vi "Get Item IO.vi"(8 "error in (no error)":errorcluster, 10 "Item Type":enum16{"RSI Module", "User Variables"}(ring), 11 "Item Ref in":T3 format="%.0x") -> (0 "error out":errorcluster, 1 "Output Data":T9 {"BD Refs"."Data Reference" format="%.0x"}, 2 "Input Data":T6 {"BD Refs"."Data Reference" format="%.0x"}, 3 "Item Ref out":T3 format="%.0x", 4 "Mixed IO":T1, 5 "To FPGA":T2[](array[typedef]) {"VS ref" format="%.0x"}, 7 "From FPGA":T2[](array[typedef]) {"VS ref" format="%.0x"})   [LabVIEW 2016, in "Scan Engine Custom Device.lvlib"]
uses:
  Scan Engine Custom Device.lvlib
  Type Defs/Output Data.ctl
  <vilib>/NI Veristand/Custom Device API/Block Data Reference.ctl
  <vilib>/NI Veristand/Custom Device API/Data Reference.ctl
  Type Defs/Input Data.ctl
  <vilib>/NI Veristand/Custom Device API/Custom Device Item Ref.ctl
  Type Defs/UDV Data.ctl
  Type Defs/UDV Data Type.ctl
  Type Defs/FXP Config.ctl
  Type Defs/Mixed IO.ctl
  Type Defs/Data Ref FGV Command.ctl
  <vilib>/NI Veristand/Custom Device API/Custom Device API.lvlib
  <vilib>/NI_Real-Time Target Support.lvlib
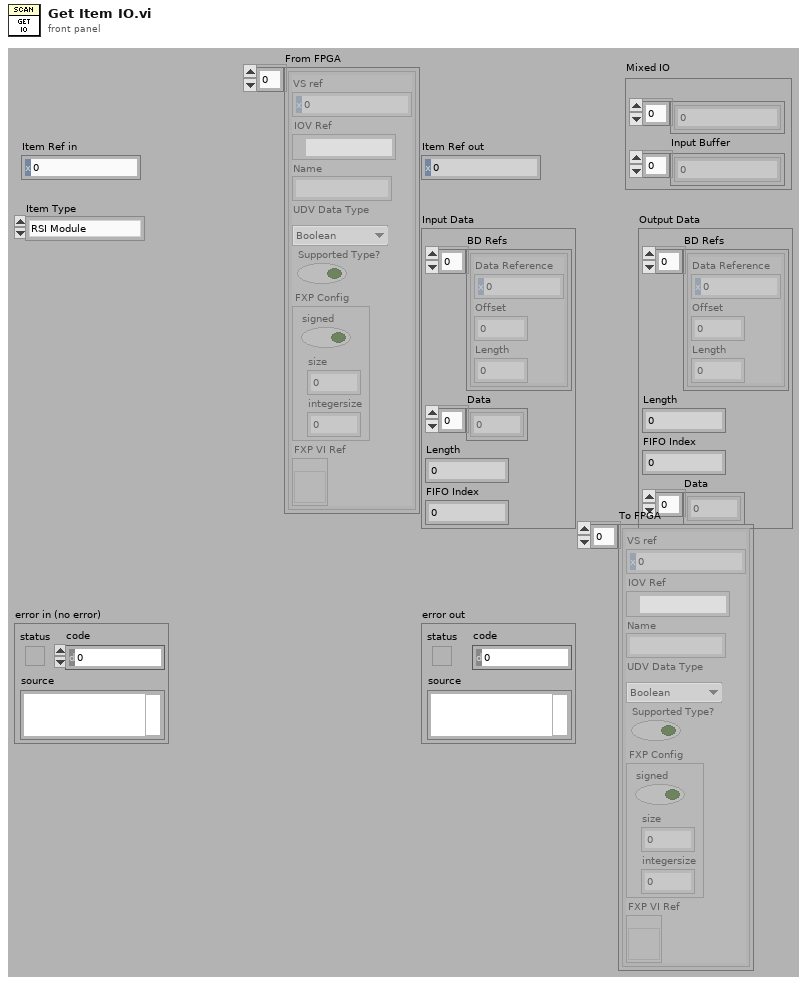
[diagram p1: front panel]
types:
  T1 = typedef "Scan Engine Custom Device.lvlib/Mixed IO.ctl" = cluster{"Input Channel Indices":i32[], "Input Buffer":dbl[]}
  T2 = typedef "Scan Engine Custom Device.lvlib/UDV Data.ctl" = cluster{"VS ref":T3, "IOV Ref":refnum<k21>, "Name":string, "UDV Data Type":T4, "Supported Type?":bool, "FXP Config":T5, "FXP VI Ref":refnum<vi>}
  T3 = typedef "Custom Device API.lvlib/Custom Device Item Ref.ctl" = u64
  T4 = typedef "Scan Engine Custom Device.lvlib/UDV Data Type.ctl" = enum16{"Boolean", "Fixed Point", "Int8", "Int16", "Int32", "Int64", "U32 Bit Field", "UInt8", "UInt16", "UInt32", "UInt64", "Other"}
  T5 = typedef "Scan Engine Custom Device.lvlib/FXP Config.ctl" = cluster{"signed":bool, "size":u32, "integersize":i32}
  T6 = typedef "Scan Engine Custom Device.lvlib/Input Data.ctl" = cluster{"BD Refs":T7[], "Data":dbl[], "Length":i32, "FIFO Index":i32}
  T7 = typedef "Custom Device API.lvlib/Block Data Reference.ctl" = cluster{"Data Reference":T8, "Offset":u64, "Length":u64}
  T8 = typedef "Custom Device API.lvlib/Data Reference.ctl" = i32
  T9 = typedef "Scan Engine Custom Device.lvlib/Output Data.ctl" = cluster{"BD Refs":T7[], "Length":i32, "FIFO Index":i32, "Data":dbl[]}
  T10 = typedef "Scan Engine Custom Device.lvlib/Data Ref FGV Command.ctl" = enum16{"Intialize", "Get", "Update"}
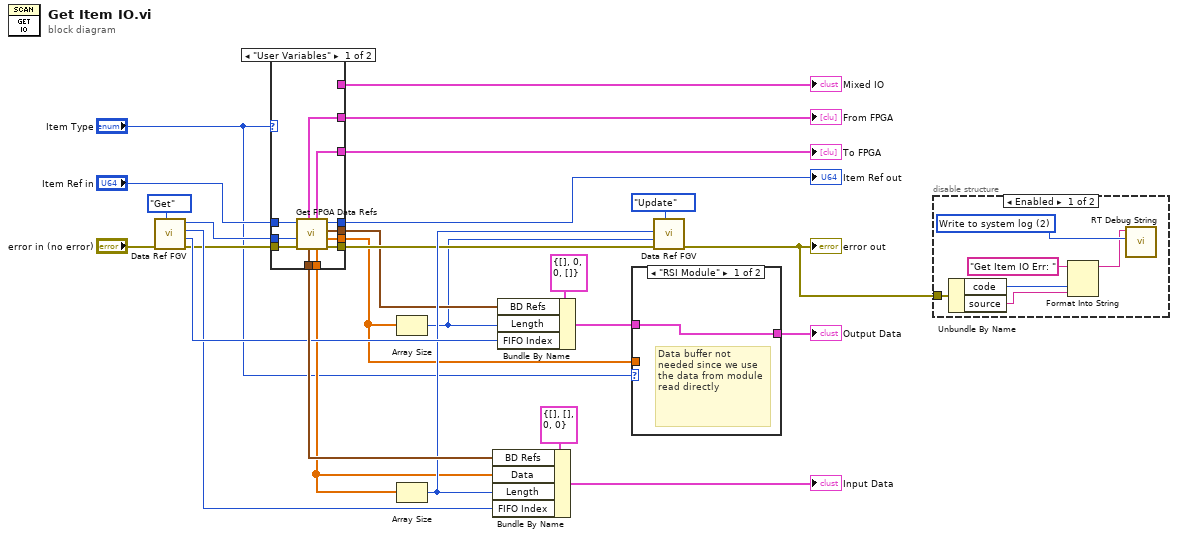
[diagram p0: block diagram]
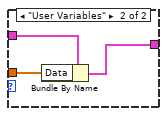
[diagram p3: hidden frame]
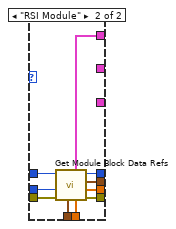
[diagram p4: hidden frame]
diagram:
  n1 = call "Data Ref FGV.vi"("Command"=Data_Ref_FGV_Command."Get", "error in (no error)"="error in (no error)") -> ("error out"=w17:errorcluster, "Output FIFO Index / Length"=w22:i32, "Input FIFO Index / Length"=w21:i32, "Device Ref out"=w12:T3)  [unwired: 6 in]
  n2 = case shown="\"User Variables\"" "Item Type" {
    tunnel: [w33 w47] -> w9
    tunnel: [w34 w46] -> w23
    tunnel: [w32 w45] -> w18
    tunnel: w17 -> [w36 w44]
    tunnel: [w30 w43] -> w15
    tunnel: [w31 w42] -> w2
    tunnel: [w29 w41] -> w14
    tunnel: "Item Ref in" -> [w37 w40]
    tunnel: w12 -> [w35 w39]
    tunnel: [w28 _] -> w8
    tunnel: [w27 _] -> w7
    tunnel: [_ w38] -> w6
    frame "User Variables" {
      n3 = call "Get FPGA Data Refs.vi"("error in"=w36, "Device Ref in"=w35, "Item Ref in"=w37) -> ("error out"=w32:errorcluster, "Output Data"=w31:dbl[], "Output Block Data Refs"=w30:T7[], "Item Ref out"=w29:T3, "Input Data"=w33:dbl[], "To FPGA"=w27:T2[], "Input Block Data Refs"=w34:T7[], "From FPGA"=w28:T2[])  [unwired: 1 in]
    }
    frame "RSI Module" {
      n4 = call "Get Module Block Data Refs.vi"("error in"=w44, "Device Ref in"=w39, "Item Ref in"=w40) -> ("error out"=w45:errorcluster, "Output Data"=w42:dbl[], "Output Block Data Refs"=w43:T7[], "Item Ref out"=w41:T3, "Input Data"=w47:dbl[], "Mixed IO"=w38:T1, "Input Block Data Refs"=w46:T7[])  [unwired: 2 in]
    }
  }
  "Item Ref out" <- w14
  "From FPGA" <- w8
  "To FPGA" <- w7
  "Mixed IO" <- w6
  n5 = Array Size(array=w2) -> (size(s)=w10:i32)
  n6 = Array Size(array=w9) -> (size(s)=w20:i32)
  n7 = Bundle By Name(cluster=T6 {"BD Refs"=[], "Data"=[], "Length"=0, "FIFO Index"=0} ("Input Data"), "BD Refs"=w23, "Data"=w9, "Length"=w20, "FIFO Index"=w21) -> (→"Input Data":T6)
  n8 = Bundle By Name(cluster=T9 {"BD Refs"=[], "Length"=0, "FIFO Index"=0, "Data"=[]} ("Output Data"), "BD Refs"=w15, "Length"=w10, "FIFO Index"=w22) -> (w4:T9)
  n9 = case shown="\"RSI Module\"" "Item Type" {
    tunnel: w4 -> [w48 w51]
    tunnel: [w48 w50] -> w3
    tunnel: w2 -> [_ w49]
    frame "RSI Module" {
      # "Data buffer not needed since we use the data from module read directly"
    }
    frame "User Variables" {
      n10 = Bundle By Name(cluster=w51, "Data"=w49) -> (w50:T9)
    }
  }
  "Output Data" <- w3
  n11 = call "Data Ref FGV.vi"("Command"=Data_Ref_FGV_Command."Update", "error in (no error)"=w18, "Output Length"=w10, "Input Length"=w20) -> ("error out"=w1:errorcluster)  [unwired: 4 in, 3 out]
  "error out" <- w1
  n12 = disable-structure shown="Enabled" {
    disable-tunnel: w1 -> [w52 _]
    frame Enabled {
      w57 = u16 2 items=["Write to serial", "Write to monitor", "Write to system log"] ("Interface")
      n13 = Unbundle By Name(w52) -> ("code"=w55:i32, "source"=w54:string)
      n14 = Format Into String(initial string="Get Item IO Err: ", w55, w54) -> (resulting string=w53:string)  [unwired: 2 in, 1 out]
      n15 = call <vilib>:"RT Debug String.vi"("Interface"=w57, "String to write"=w53) -> ()  [unwired: 9 in, 1 out]
    }
    frame Disabled {
    }
  }
